vi "Variant_GetType.vi"(11 "Variant":variant) -> (1 "LV Type Enum":T1 format="%02x", 2 "Type":u8 format="%.0x", 3 "Variant dup":variant)   [LabVIEW 2013, in "OpenVariant.lvlib"]
uses:
  OpenVariant.lvlib
  <vilib>/Utility/VariantDataType/Type.ctl
  TypeDescriptor/OpenDescriptor.lvlib
  <vilib>/Utility/VariantDataType/VariantType.lvlib
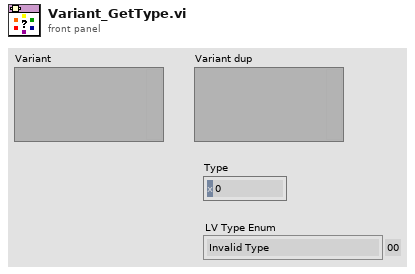
[diagram p1: front panel]
types:
  T1 = typedef "VariantType.lvlib/Type.ctl" = enum8{"Invalid Type", "Void", "I8", "I16", "I32", "I64", "U8", "U16", "U32", "U64", "Single Float", "Double Float", "Extended Float", "Single Complex", "Double Complex", "Extended Complex", "Enum U8", "Enum U16", "Enum U32", "Enum U64", "Single Float With Unit", "Double Float With Unit", "Extended Float With Unit", "Single Complex with Unit", "Double Complex with Unit", "Extended Complex with Unit", "Boolean", "String", "Path", "Picture", "Tag", "Array", "Cluster", "Variant", "LV Variant", "Waveform", "Timestamp", "Digital Waveform", "Digital Data", "ExpressData", "Refnum", "External Data", "VI", "Poly VI", "LabVIEW Class Instance", "Fixed Point"}
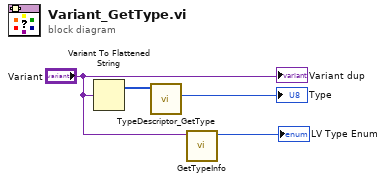
[diagram p0: block diagram]
diagram:
  n1 = Variant To Flattened String(Variant="Variant") -> (1:w4:i16[])  [unwired: 1 out]
  n2 = call "TypeDescriptor_GetType.vi"("type descriptor"=w4) -> ("Type"=→"Type":u8)  [unwired: 9 in, 1 out]
  n3 = call <vilib>:"GetTypeInfo.vi"("Variant"="Variant") -> ("Type Enum"=→"LV Type Enum":T1)  [unwired: 6 in, 4 out]
  "Variant dup" <- "Variant"
